vi "random_colour.vi"(1 "string in":string) -> (0 "string out, with %%randcol%% replaced with a 4-element colour":string)   [LabVIEW 2010]
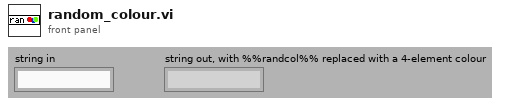
[diagram p1: front panel]
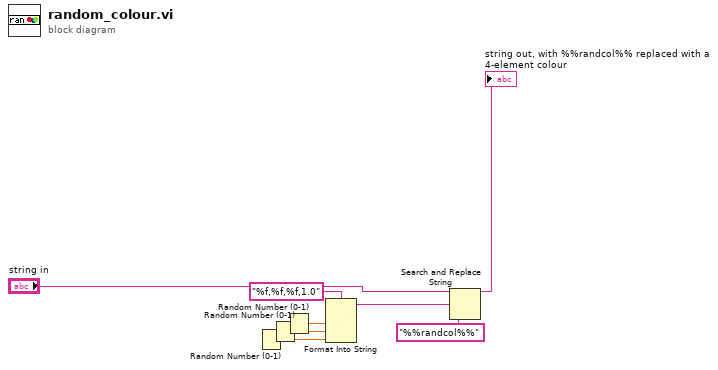
[diagram p0: block diagram]
diagram:
  n1 = Random Number (0-1)() -> (number: 0 to 1=w3:dbl)
  n2 = Random Number (0-1)() -> (number: 0 to 1=w2:dbl)
  n3 = Random Number (0-1)() -> (number: 0 to 1=w1:dbl)
  n4 = Format Into String(format string="%f,%f,%f,1.0", w1, w2, w3) -> (resulting string=w7:string)  [unwired: 2 in, 1 out]
  n5 = Search and Replace String(input string="string in", search string="%%randcol%%", replace string=w7) -> (result string=→"string out, with %%randcol%% replaced with a 4-element colour":string)  [unwired: 5 in, 3 out]
